vi "Keithley 2600 Series Read Current Measurement.vi"() -> ()   [LabVIEW 2019, in "Keithley 2600 Series.lvlib"]
doc: "This example shows how to configure the source output and perform multiple current measurements."
uses:
  Public/Configure/Source/Configure Source (Range).vi
  Public/Configure/Source/Configure Source (Level).vi
  Public/Configure/Source/Configure Source (Limit).vi
  Public/Data/Read Measurement (Current).vi
  Keithley 2600 Series.lvlib
panel:
  out "Current Buffer Data (A)":dbl[](array[numeric])
  in  "Measurement Count (10)":i32=10
  in  "Current Limit (0.1 A)":dbl=0.1
  in  "Voltage Level (1 V)":dbl=1.0
  in  "Source Function (1: Voltage)":i32(ring)=1 items=["Voltage"=1]
  in  "Source Measure Unit Channel (0: Channel A)":i32(ring) items=["Channel A", "Channel B"]
  in  "VISA resource name":refnum<visa-resource-name>
  # "(c) 2020 - 2022 National Instruments.  ALL RIGHTS RESERVED."
  # "Source Output Configuration"
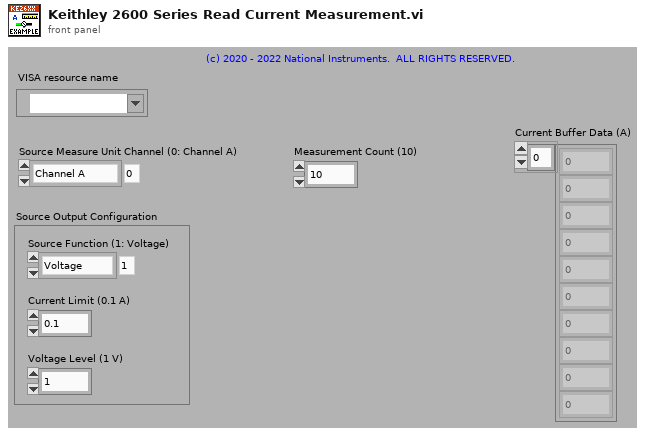
[diagram p1: front panel]
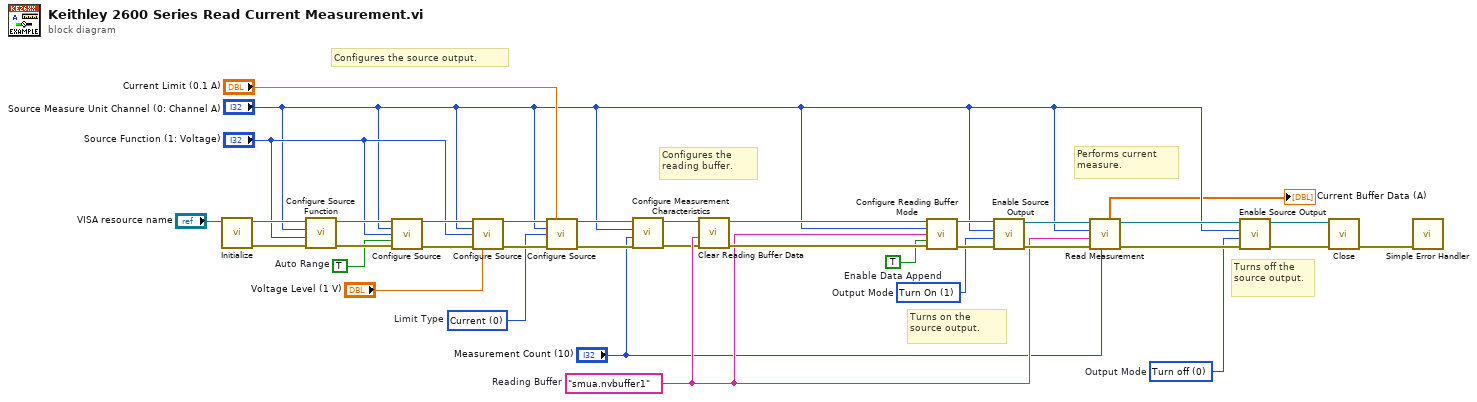
[diagram p0: block diagram]
diagram:
  w1 = 0 items=["Current", "Voltage", "Power"]  # Limit Type
  w12 = 0 items=["Turn off", "Turn On", "High-Z"]  # Output Mode
  w18 = 1 items=["Turn off", "Turn On", "High-Z"]  # Output Mode
  w21 = TRUE  # Enable Data Append
  w15 = "smua.nvbuffer1"  # Reading Buffer
  w29 = TRUE  # Auto Range
  # "Turns on the source output."
  # "Configures the reading buffer."
  # "Configures the source output."
  # "Performs current measure."
  # "Turns off the source output."
  n1 = call "Initialize.vi"("VISA resource name"="VISA resource name") -> ("error out"=w34:errorcluster, "VISA resource name out"=w35:refnum<visa-resource-name>)  [unwired: 9 in]
  n2 = call "Configure Source Function.vi"("error in (no error)"=w34, "Source Function (1: Voltage)"="Source Function (1: Voltage)", "Source Measure Unit Channel (0: Channel A)"="Source Measure Unit Channel (0: Channel A)", "VISA resource name"=w35) -> ("error out"=w32:errorcluster, "VISA resource name out"=w33:refnum<visa-resource-name>)  [unwired: 6 in]
  n3 = call-poly "Configure Source.vi"("VISA resource name"=w33, "Source Measure Unit Channel (0: Channel A)"="Source Measure Unit Channel (0: Channel A)", "Range Type (1: Voltage)"="Source Function (1: Voltage)", "Auto Range (T: Enable)"=w29, "error in (no error)"=w32) -> ("VISA resource name out"=w31:refnum<visa-resource-name>, "error out"=w30:errorcluster)  [unwired: 9 in]
  n4 = call-poly "Configure Source.vi"("VISA resource name"=w31, "Source Measure Unit Channel (0: Channel A)"="Source Measure Unit Channel (0: Channel A)", "Level Type (1: Voltage)"="Source Function (1: Voltage)", "error in (no error)"=w30, "Voltage Level (0 V)"="Voltage Level (1 V)") -> ("VISA resource name out"=w27:refnum<visa-resource-name>, "error out"=w26:errorcluster)  [unwired: 9 in]
  n5 = call-poly "Configure Source.vi"("VISA resource name"=w27, "Current Limit (0.1 A)"="Current Limit (0.1 A)", "Source Measure Unit Channel (0: Channel A)"="Source Measure Unit Channel (0: Channel A)", "Limit Type (1: Voltage)"=w1, "error in (no error)"=w26) -> ("VISA resource name out"=w11:refnum<visa-resource-name>, "error out"=w10:errorcluster)  [unwired: 9 in]
  n6 = call "Configure Measurement Characteristics.vi"("error in (no error)"=w10, "Measurement Count (1)"="Measurement Count (10)", "Source Measure Unit Channel (0: Channel A)"="Source Measure Unit Channel (0: Channel A)", "VISA resource name"=w11) -> ("error out"=w8:errorcluster, "VISA resource name out"=w9:refnum<visa-resource-name>)  [unwired: 6 in]
  n7 = call "Clear Reading Buffer Data.vi"("error in (no error)"=w8, "Reading Buffer (smua.nvbuffer1)"=w15, "VISA resource name"=w9) -> ("error out"=w22:errorcluster, "VISA resource name out"=w23:refnum<visa-resource-name>)  [unwired: 7 in]
  n8 = call "Configure Reading Buffer Mode.vi"("VISA resource name"=w23, "Source Measure Unit Channel (0: Channel A)"="Source Measure Unit Channel (0: Channel A)", "Reading Buffer (smua.nvbuffer1)"=w15, "Enable Data Append (F: Disable)"=w21, "error in (no error)"=w22) -> ("VISA resource name out"=w20:refnum<visa-resource-name>, "error out"=w19:errorcluster)  [unwired: 9 in]
  n9 = call "Enable Source Output.vi"("error in (no error)"=w19, "Output Mode (0: Turn off)"=w18, "Source Measure Unit Channel (0: Channel A)"="Source Measure Unit Channel (0: Channel A)", "VISA resource name"=w20) -> ("error out"=w16:errorcluster, "VISA resource name out"=w17:refnum<visa-resource-name>)  [unwired: 6 in]
  n10 = call-poly "Read Measurement.vi"("Wait Time (10 S)"="Measurement Count (10)", "error in (no error)"=w16, "Current Buffer (smua.nvbuffer1)"=w15, "Source Measure Unit Channel (0: Channel A)"="Source Measure Unit Channel (0: Channel A)", "VISA resource name"=w17) -> ("error out"=w13:errorcluster, "VISA resource name out"=w14:refnum<visa-resource-name>, "Current Buffer Data (A)"=→"Current Buffer Data (A)":dbl[])  [unwired: 3 in, 1 out]
  n11 = call "Enable Source Output.vi"("error in (no error)"=w13, "Output Mode (0: Turn off)"=w12, "Source Measure Unit Channel (0: Channel A)"="Source Measure Unit Channel (0: Channel A)", "VISA resource name"=w14) -> ("error out"=w3:errorcluster, "VISA resource name out"=w4:refnum<visa-resource-name>)  [unwired: 6 in]
  n12 = call "Close.vi"("error in (no error)"=w3, "VISA resource name"=w4) -> ("error out"=w2:errorcluster)  [unwired: 9 in]
  n13 = call <vilib>:"Simple Error Handler.vi"("error in (no error)"=w2) -> ()  [unwired: 4 in, 5 out]
